vi "my_read_data.vi"() -> ()   [LabVIEW 2020]
panel:
  in  "基路径":path
  # "外部自定义轨迹读取程序"
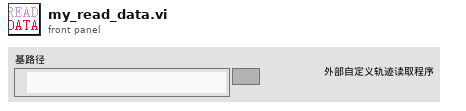
[diagram p1: front panel]
types:
  T1 = enum16{"big-endian, network order", "native, host order", "little-endian"}
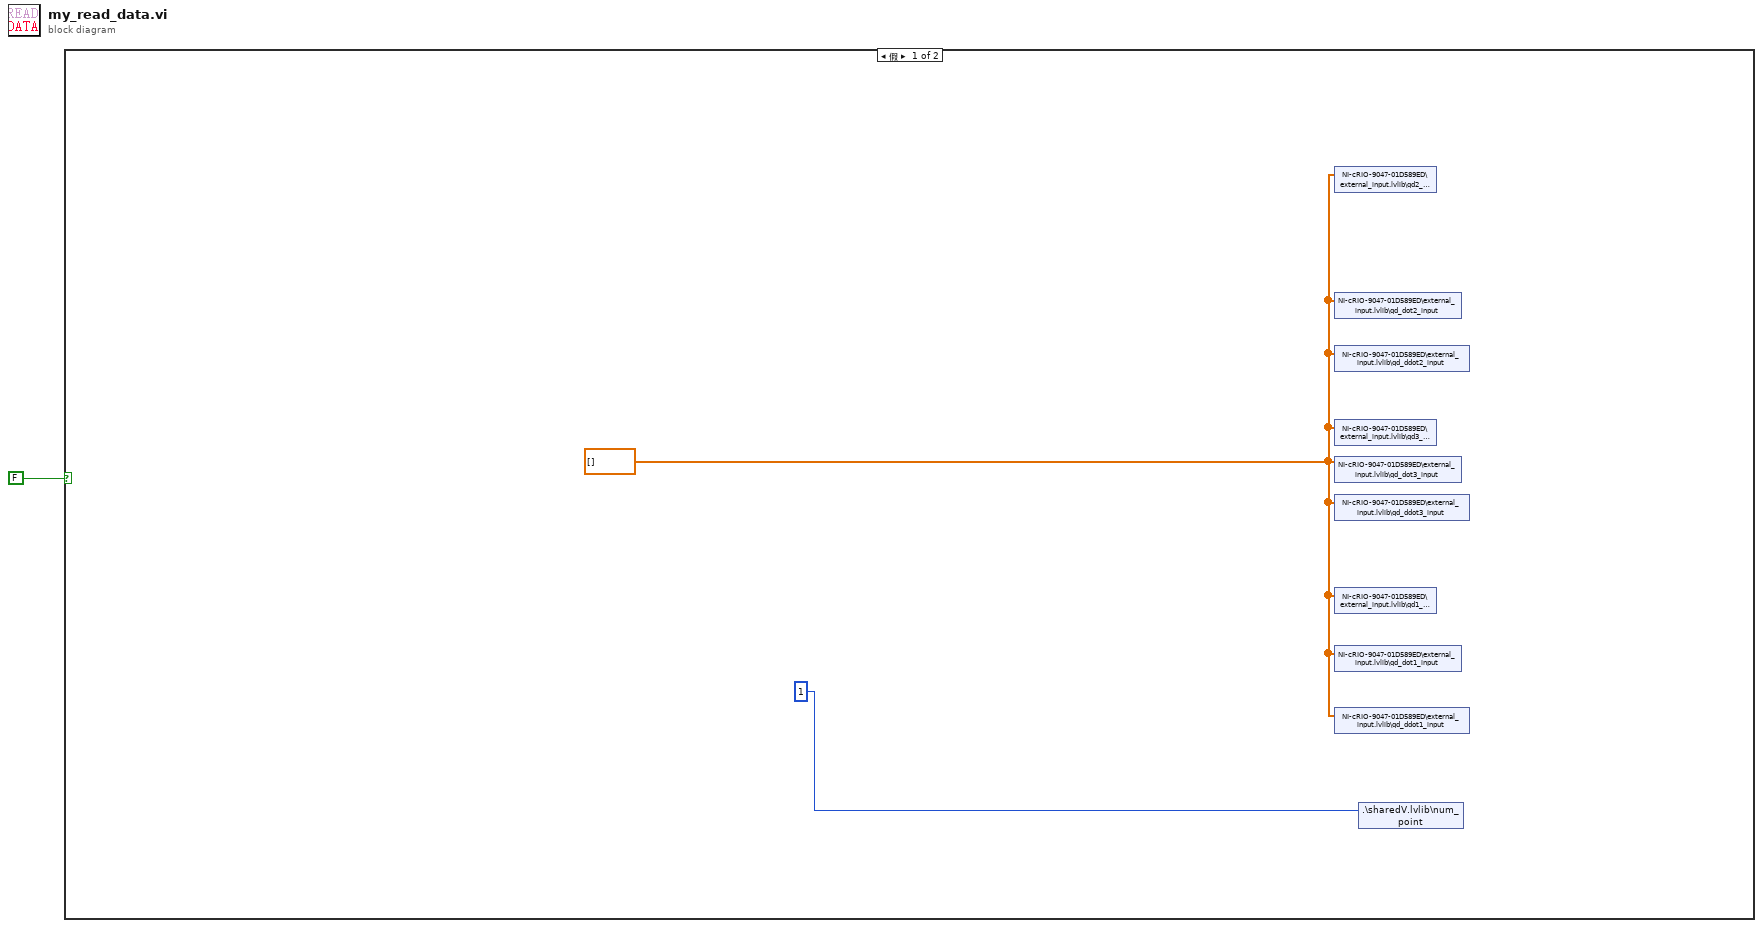
[diagram p0: block diagram]
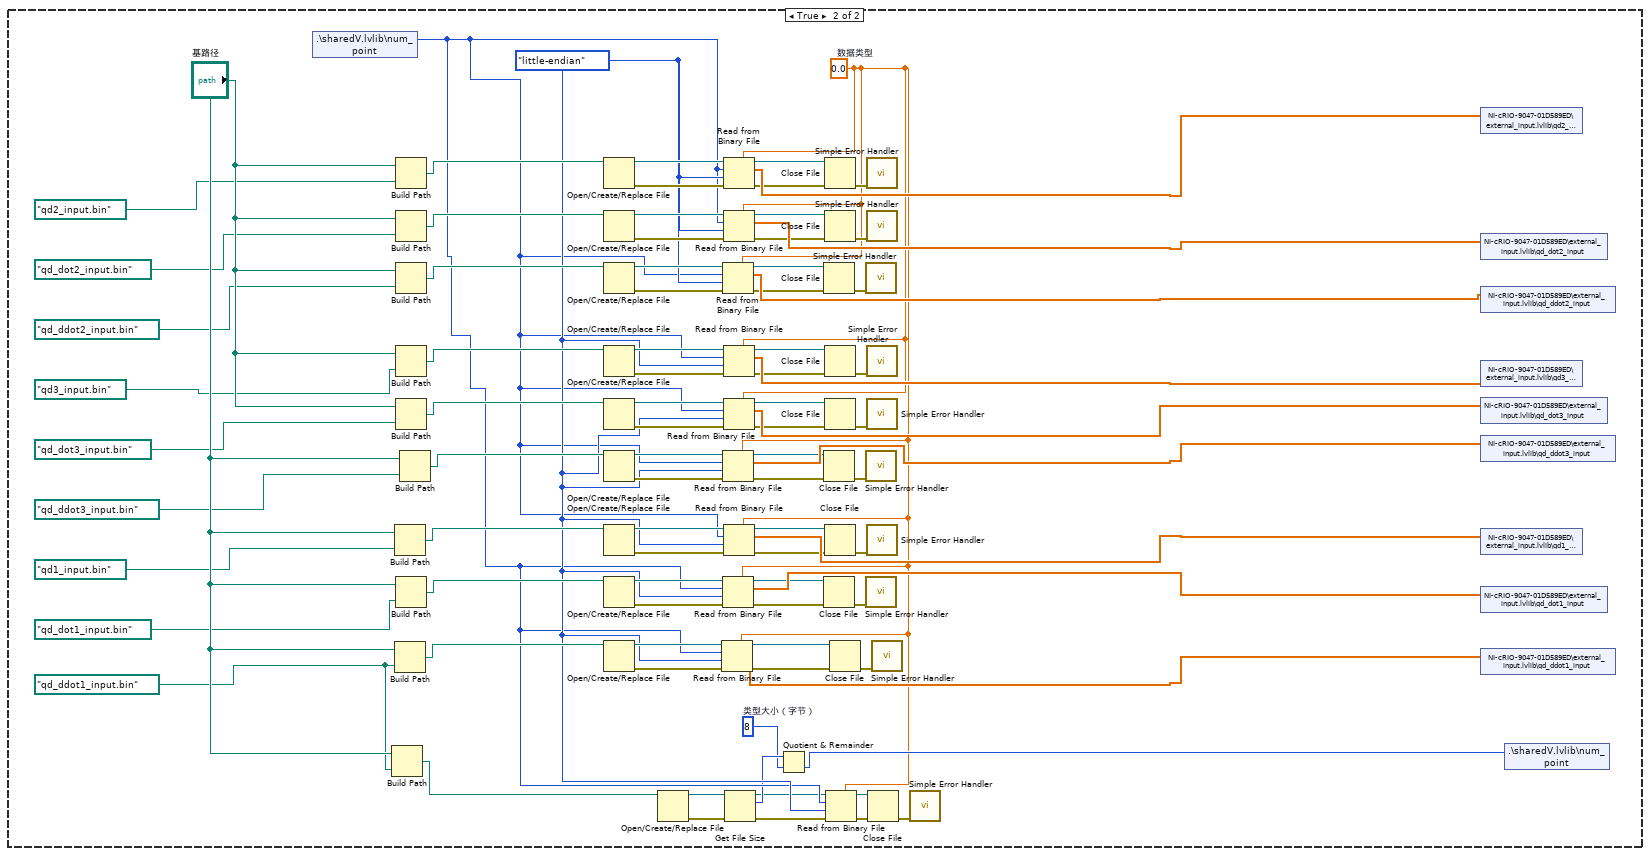
[diagram p2: hidden frame]
diagram:
  n1 = case shown="假" FALSE {
    frame False {
      w2 = dbl[] []
      n2 = shared-variable "NI-cRIO-9047-01D589ED\\external_input.lvlib\\qd2_input"(w2) -> ()  [unwired: 1 in, 1 out]
      n3 = shared-variable "NI-cRIO-9047-01D589ED\\external_input.lvlib\\qd_dot2_input"(w2) -> ()  [unwired: 1 in, 1 out]
      n4 = shared-variable "NI-cRIO-9047-01D589ED\\external_input.lvlib\\qd_ddot2_input"(w2) -> ()  [unwired: 1 in, 1 out]
      n5 = shared-variable "NI-cRIO-9047-01D589ED\\external_input.lvlib\\qd3_input"(w2) -> ()  [unwired: 1 in, 1 out]
      n6 = shared-variable "NI-cRIO-9047-01D589ED\\external_input.lvlib\\qd_dot3_input"(w2) -> ()  [unwired: 1 in, 1 out]
      n7 = shared-variable "NI-cRIO-9047-01D589ED\\external_input.lvlib\\qd_ddot3_input"(w2) -> ()  [unwired: 1 in, 1 out]
      n8 = shared-variable "NI-cRIO-9047-01D589ED\\external_input.lvlib\\qd1_input"(w2) -> ()  [unwired: 1 in, 1 out]
      n9 = shared-variable "NI-cRIO-9047-01D589ED\\external_input.lvlib\\qd_dot1_input"(w2) -> ()  [unwired: 1 in, 1 out]
      n10 = shared-variable "NI-cRIO-9047-01D589ED\\external_input.lvlib\\qd_ddot1_input"(w2) -> ()  [unwired: 1 in, 1 out]
      n11 = shared-variable ".\\sharedV.lvlib\\num_point"(1) -> ()  [unwired: 1 in, 1 out]
    }
    frame True {
      w5 = i64 8  # 类型大小（字节）
      w17 = 0.0  # 数据类型
      w16 = T1."little-endian" ("字节顺序(0:big-endian, network order)")
      w4 = path "qd_ddot1_input.bin" ("file path (use dialog)")
      n12 = shared-variable ".\\sharedV.lvlib\\num_point"() -> (w15:i32)  [unwired: 1 in, 1 out]
      n13 = Build Path(base path="基路径", name or relative path=w4) -> (appended path=w14:path)
      n14 = Build Path(base path="基路径", name or relative path=path "qd1_input.bin" ("file path (use dialog)")) -> (appended path=w72:path)
      n15 = Build Path(base path="基路径", name or relative path=w4) -> (appended path=w74:path)
      n16 = Build Path(base path="基路径", name or relative path=path "qd2_input.bin" ("file path (use dialog)")) -> (appended path=w66:path)
      n17 = Build Path(base path="基路径", name or relative path=path "qd_dot2_input.bin" ("file path (use dialog)")) -> (appended path=w67:path)
      n18 = Build Path(base path="基路径", name or relative path=path "qd_ddot2_input.bin" ("file path (use dialog)")) -> (appended path=w68:path)
      n19 = Build Path(base path="基路径", name or relative path=path "qd3_input.bin" ("file path (use dialog)")) -> (appended path=w69:path)
      n20 = Build Path(base path="基路径", name or relative path=path "qd_dot3_input.bin" ("file path (use dialog)")) -> (appended path=w70:path)
      n21 = Build Path(base path="基路径", name or relative path=path "qd_dot1_input.bin" ("file path (use dialog)")) -> (appended path=w73:path)
      n22 = Build Path(base path="基路径", name or relative path=path "qd_ddot3_input.bin" ("file path (use dialog)")) -> (appended path=w71:path)
      n23 = Open/Create/Replace File(file path (use dialog)=w66) -> (refnum out=w29:refnum<file>, error out=w28:errorcluster)  [unwired: 5 in, 1 out]
      n24 = Open/Create/Replace File(file path (use dialog)=w67) -> (refnum out=w34:refnum<file>, error out=w33:errorcluster)  [unwired: 5 in, 1 out]
      n25 = Open/Create/Replace File(file path (use dialog)=w68) -> (refnum out=w39:refnum<file>, error out=w38:errorcluster)  [unwired: 5 in, 1 out]
      n26 = Open/Create/Replace File(file path (use dialog)=w69) -> (refnum out=w44:refnum<file>, error out=w43:errorcluster)  [unwired: 5 in, 1 out]
      n27 = Open/Create/Replace File(file path (use dialog)=w70) -> (refnum out=w49:refnum<file>, error out=w48:errorcluster)  [unwired: 5 in, 1 out]
      n28 = Open/Create/Replace File(file path (use dialog)=w71) -> (refnum out=w54:refnum<file>, error out=w53:errorcluster)  [unwired: 5 in, 1 out]
      n29 = Open/Create/Replace File(file path (use dialog)=w72) -> (refnum out=w64:refnum<file>, error out=w58:errorcluster)  [unwired: 5 in, 1 out]
      n30 = Open/Create/Replace File(file path (use dialog)=w73) -> (refnum out=w62:refnum<file>, error out=w61:errorcluster)  [unwired: 5 in, 1 out]
      n31 = Open/Create/Replace File(file path (use dialog)=w74) -> (refnum out=w75:refnum<file>, error out=w76:errorcluster)  [unwired: 5 in, 1 out]
      n32 = Open/Create/Replace File(file path (use dialog)=w14) -> (refnum out=w10:refnum<file>, error out=w8:errorcluster)  [unwired: 5 in, 1 out]
      n33 = Read from Binary File(5:w17, 8:w76, 9:w16, 10:w15, 11:w75) -> (0:w79:errorcluster, 2:w90:dbl[], 3:w78:refnum<file>)  [unwired: 1 in, 1 out]
      n34 = Read from Binary File(5:w17, 8:w38, 9:w16, 10:w15, 11:w39) -> (0:w36:errorcluster, 2:w84:dbl[], 3:w40:refnum<file>)  [unwired: 1 in, 1 out]
      n35 = Read from Binary File(5:w17, 8:w53, 9:w16, 10:w15, 11:w54) -> (0:w51:errorcluster, 2:w87:dbl[], 3:w55:refnum<file>)  [unwired: 1 in, 1 out]
      n36 = Read from Binary File(5:w17, 8:w61, 9:w16, 10:w15, 11:w62) -> (0:w59:errorcluster, 2:w89:dbl[], 3:w63:refnum<file>)  [unwired: 1 in, 1 out]
      n37 = Read from Binary File(5:w17, 8:w28, 9:w16, 10:w15, 11:w29) -> (0:w26:errorcluster, 2:w82:dbl[], 3:w30:refnum<file>)  [unwired: 1 in, 1 out]
      n38 = Read from Binary File(5:w17, 8:w33, 9:w16, 10:w15, 11:w34) -> (0:w31:errorcluster, 2:w83:dbl[], 3:w35:refnum<file>)  [unwired: 1 in, 1 out]
      n39 = Read from Binary File(5:w17, 8:w43, 9:w16, 10:w15, 11:w44) -> (0:w41:errorcluster, 2:w85:dbl[], 3:w45:refnum<file>)  [unwired: 1 in, 1 out]
      n40 = Read from Binary File(5:w17, 8:w48, 9:w16, 10:w15, 11:w49) -> (0:w46:errorcluster, 2:w86:dbl[], 3:w50:refnum<file>)  [unwired: 1 in, 1 out]
      n41 = Read from Binary File(5:w17, 8:w58, 9:w16, 10:w15, 11:w64) -> (0:w56:errorcluster, 2:w88:dbl[], 3:w65:refnum<file>)  [unwired: 1 in, 1 out]
      n42 = Get File Size(file=w10, error in=w8) -> (refnum out=w11:refnum<file>, size (in bytes)=w12:i64, 0:w7:errorcluster)
      n43 = Quotient & Remainder(x=w12, y=w5) -> (floor(x/y)=w81:i64)  [unwired: 1 out]
      n44 = Close File(refnum=w40, error in=w36) -> (error out=w37:errorcluster)  [unwired: 1 out]
      n45 = Close File(refnum=w55, error in=w51) -> (error out=w52:errorcluster)  [unwired: 1 out]
      n46 = Close File(refnum=w63, error in=w59) -> (error out=w60:errorcluster)  [unwired: 1 out]
      n47 = Close File(refnum=w30, error in=w26) -> (error out=w27:errorcluster)  [unwired: 1 out]
      n48 = Close File(refnum=w35, error in=w31) -> (error out=w32:errorcluster)  [unwired: 1 out]
      n49 = Close File(refnum=w45, error in=w41) -> (error out=w42:errorcluster)  [unwired: 1 out]
      n50 = Close File(refnum=w50, error in=w46) -> (error out=w47:errorcluster)  [unwired: 1 out]
      n51 = Close File(refnum=w65, error in=w56) -> (error out=w57:errorcluster)  [unwired: 1 out]
      n52 = Read from Binary File(5:w17, 8:w7, 9:w16, 10:w15, 11:w11) -> (0:w6:errorcluster, 3:w13:refnum<file>)  [unwired: 1 in, 2 out]
      n53 = Close File(refnum=w78, error in=w79) -> (error out=w77:errorcluster)  [unwired: 1 out]
      n54 = call <vilib>:"Simple Error Handler.vi"("error in (no error)"=w37) -> ()  [unwired: 4 in, 5 out]
      n55 = call <vilib>:"Simple Error Handler.vi"("error in (no error)"=w52) -> ()  [unwired: 4 in, 5 out]
      n56 = call <vilib>:"Simple Error Handler.vi"("error in (no error)"=w60) -> ()  [unwired: 4 in, 5 out]
      n57 = call <vilib>:"Simple Error Handler.vi"("error in (no error)"=w27) -> ()  [unwired: 4 in, 5 out]
      n58 = call <vilib>:"Simple Error Handler.vi"("error in (no error)"=w32) -> ()  [unwired: 4 in, 5 out]
      n59 = call <vilib>:"Simple Error Handler.vi"("error in (no error)"=w42) -> ()  [unwired: 4 in, 5 out]
      n60 = call <vilib>:"Simple Error Handler.vi"("error in (no error)"=w47) -> ()  [unwired: 4 in, 5 out]
      n61 = call <vilib>:"Simple Error Handler.vi"("error in (no error)"=w57) -> ()  [unwired: 4 in, 5 out]
      n62 = Close File(refnum=w13, error in=w6) -> (error out=w9:errorcluster)  [unwired: 1 out]
      n63 = call <vilib>:"Simple Error Handler.vi"("error in (no error)"=w77) -> ()  [unwired: 4 in, 5 out]
      n64 = call <vilib>:"Simple Error Handler.vi"("error in (no error)"=w9) -> ()  [unwired: 4 in, 5 out]
      n65 = shared-variable "NI-cRIO-9047-01D589ED\\external_input.lvlib\\qd2_input"(w82) -> ()  [unwired: 1 in, 1 out]
      n66 = shared-variable "NI-cRIO-9047-01D589ED\\external_input.lvlib\\qd_dot2_input"(w83) -> ()  [unwired: 1 in, 1 out]
      n67 = shared-variable "NI-cRIO-9047-01D589ED\\external_input.lvlib\\qd_ddot2_input"(w84) -> ()  [unwired: 1 in, 1 out]
      n68 = shared-variable "NI-cRIO-9047-01D589ED\\external_input.lvlib\\qd3_input"(w85) -> ()  [unwired: 1 in, 1 out]
      n69 = shared-variable "NI-cRIO-9047-01D589ED\\external_input.lvlib\\qd_dot3_input"(w86) -> ()  [unwired: 1 in, 1 out]
      n70 = shared-variable "NI-cRIO-9047-01D589ED\\external_input.lvlib\\qd_ddot3_input"(w87) -> ()  [unwired: 1 in, 1 out]
      n71 = shared-variable "NI-cRIO-9047-01D589ED\\external_input.lvlib\\qd1_input"(w88) -> ()  [unwired: 1 in, 1 out]
      n72 = shared-variable "NI-cRIO-9047-01D589ED\\external_input.lvlib\\qd_dot1_input"(w89) -> ()  [unwired: 1 in, 1 out]
      n73 = shared-variable "NI-cRIO-9047-01D589ED\\external_input.lvlib\\qd_ddot1_input"(w90) -> ()  [unwired: 1 in, 1 out]
      n74 = shared-variable ".\\sharedV.lvlib\\num_point"(w81) -> ()  [unwired: 1 in, 1 out]
    }
  }
